vi "Untitled 1.vi"() -> ()   [LabVIEW 2013]
uses:
  <vilib>/MakerHub/LINX/Public/Peripherals/Digital/Digital Write 1 Chan.vi
  <vilib>/MakerHub/LINX/Public/Peripherals/Analog/Analog Read 1 Chan.vi
  <vilib>/MakerHub/LINX/Public/Peripherals/Digital/Digital Write N Chans.vi
  <vilib>/MakerHub/LINX/Public/Peripherals/Analog/Analog Read N Chans.vi
  <vilib>/MakerHub/LINX/Private/Local IO/LinxDigitalWrite.vi
  <vilib>/MakerHub/LINX/Public/Utilities/Check Channel.vi
  <vilib>/MakerHub/LINX/Private/Local IO/LinxAnalogRead.vi
  <vilib>/MakerHub/LINX/Public/Utilities/Open Serial.vi
  <vilib>/Utility/config.llb/Read Key (I32).vi
  <vilib>/Utility/config.llb/Read Key (Double).vi
  <vilib>/Utility/config.llb/Read Key (U32).vi
  <vilib>/Utility/config.llb/Write Key (U32).vi
  <vilib>/Utility/config.llb/Write Key (Double).vi
  <vilib>/MakerHub/LINX/Private/Utilties/Generate Error.vi
  <vilib>/express/express arith-compare/Formula/XNode/ExpressFormulaBlockNode.xnode
  <vilib>/MakerHub/LINX/LMH-LINX.lvlib
  <vilib>/Utility/config.llb/NI_LVConfig.lvlib
panel:
  out "Alarm":bool
  out "Relay":bool
  out "Moisture Value":dbl
  out "Alarm Pin":dbl
  out "Relay Pin":dbl
  out "Sensor Pin":dbl
  out "Critical Moisture Level":dbl
  out "Higher Moisture Level":dbl
  out "Lower Moisture Level":dbl
  in  "?":bool
  in  "Sensor":u8
  in  "higher moisture level":dbl
  in  "Relay":u8
  in  "critical moisture level":dbl
  in  "Alarm":u8
  in  "lower moisture level":dbl
  out "Moisture Level":dbl(slide) scale=0.0..100.0
  out "Waveform Chart":dbl(graph)
  in  "?":bool
  in  "Serial Port":refnum<visa-resource-name>="N/A"
  # "Automatic Plant Watering System"
  # "Pin Connections"
  # "Moisture Levels"
  # "Settings"
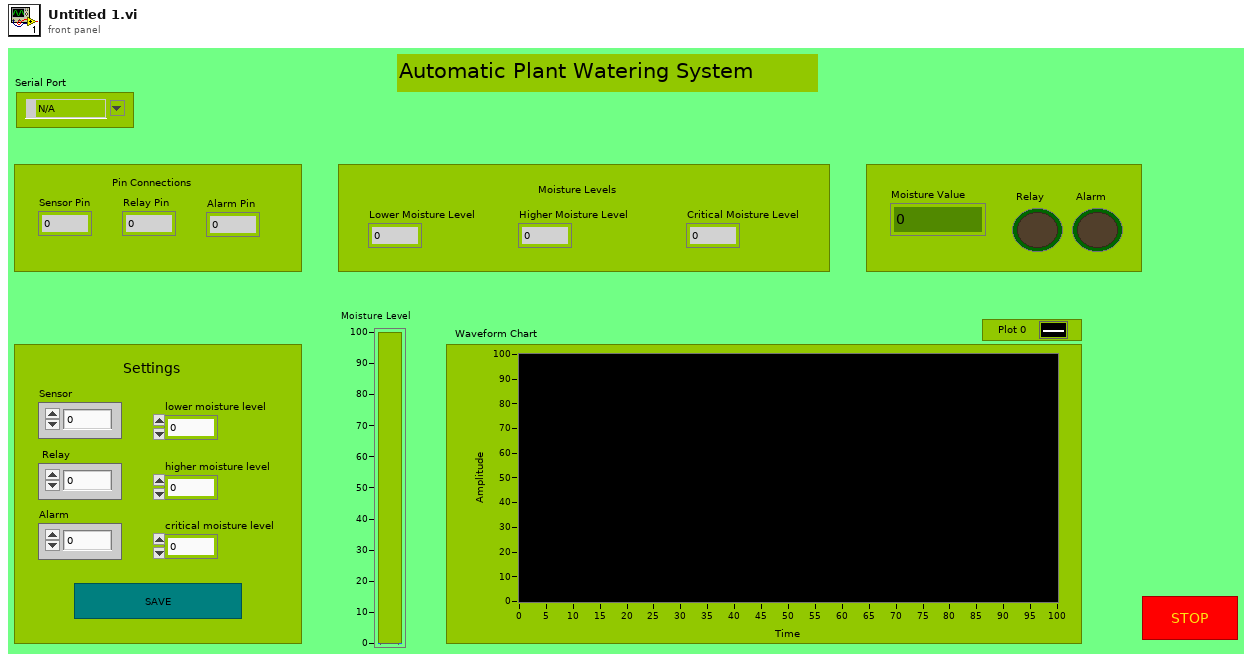
[diagram p1: front panel]
types:
  T1 = typedef "LMH-LINX.lvlib/LINX Ref.ctl" = cluster{"IO":T2, "Interface":T3, "LINX Device Config":T4}
  T2 = typedef "LMH-LINX.lvlib/Platform.ctl" = enum16{"Remote", "Local"}
  T3 = typedef "LMH-LINX.lvlib/Interface.ctl" = enum16{"Serial", "TCP"}
  T4 = typedef "LMH-LINX.lvlib/Device.lvlib/LINX Device Config.ctl" = cluster{"Interface":T3, "COM Port":refnum<visa-resource-name>, "TCP Configuration":T5, "Device Family":u8, "Device ID":u8, "Device Name":string, "TCP Ref":refnum<k5>, "Channels":T6}
  T5 = typedef "LMH-LINX.lvlib/Device.lvlib/TCP Config.ctl" = cluster{"IP Address":string, "Port":u16}
  T6 = typedef "LMH-LINX.lvlib/Channels.ctl" = cluster{"DI":u8[], "DO":u8[], "AI":u8[], "AO":u8[], "PWM":u8[], "QE":u8[], "UART":u8[], "I2C 2":u8[], "SPI":u8[], "CAN":u8[], "Servo":u8[], "AI Ref (V)":dbl, "AI Resolution (Bits)":u8, "AO Ref (V)":dbl, "AO Resolution (Bits)":u8}
  T7 = typedef "NI_LVConfig.lvlib/Config Data RefNum.ctl" = refnum<k1>
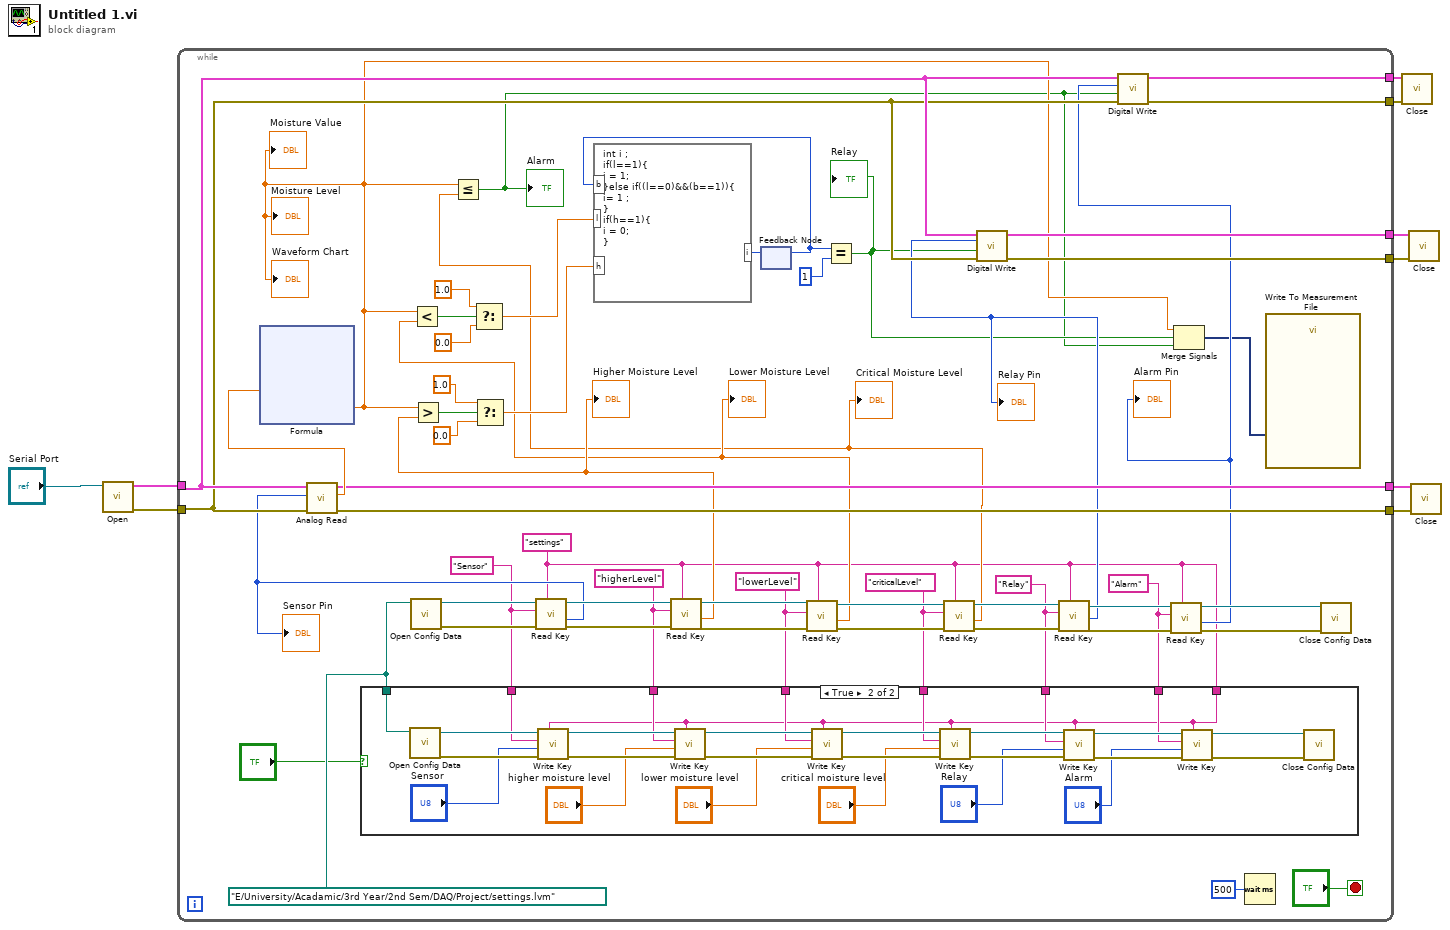
[diagram p0: block diagram]
diagram:
  n1 = call-poly <vilib>:"Open.vi"("Serial Port"="Serial Port") -> ("Error Out"=w6:errorcluster, "LINX Resource"=w7:T1)  [unwired: 8 in, 1 out]
  n2 = while {
    tunnel: [w62] -> w9
    tunnel: [w54] -> w8
    tunnel: w7 -> [w59]
    tunnel: w6 -> [w58]
    tunnel: [w61] -> w5
    tunnel: [w60] -> w4
    tunnel: [w57] -> w3
    tunnel: [w56] -> w2
    stop <- "?" stop-if-true
    w16 = "Alarm" ("key")
    w17 = "Relay" ("key")
    w18 = "criticalLevel" ("key")
    w19 = "lowerLevel" ("key")
    w20 = "higherLevel" ("key")
    w21 = "Sensor" ("key")
    w15 = "settings" ("section")
    w22 = path "E:/University/Acadamic/3rd Year/2nd Sem/DAQ/Project/settings.lvm" ("configuration file path")
    n3 = case shown="True" "?" {
      tunnel: w22 -> [_ w90]
      tunnel: w21 -> [_ w77]
      tunnel: w20 -> [_ w76]
      tunnel: w19 -> [_ w75]
      tunnel: w18 -> [_ w74]
      tunnel: w17 -> [_ w73]
      tunnel: w16 -> [_ w72]
      tunnel: w15 -> [_ w71]
      frame False {
      }
      frame True {
        n4 = call <vilib>:"Open Config Data.vi"("configuration file path"=w90) -> ("error out"=w91:errorcluster, "refnum"=w92:T7)  [unwired: 8 in, 1 out]
        n5 = call-poly <vilib>:"Write Key.vi"("section"=w71, "error in (no error)"=w91, "value"="Sensor", "key"=w77, "refnum"=w92) -> ("error out"=w88:errorcluster, "refnum out"=w89:T7)  [unwired: 4 in, 1 out]
        n6 = call-poly <vilib>:"Write Key.vi"("section"=w71, "error in (no error)"=w88, "value"="higher moisture level", "key"=w76, "refnum"=w89) -> ("error out"=w86:errorcluster, "refnum out"=w87:T7)  [unwired: 4 in, 1 out]
        n7 = call-poly <vilib>:"Write Key.vi"("section"=w71, "error in (no error)"=w86, "value"="lower moisture level", "key"=w75, "refnum"=w87) -> ("error out"=w84:errorcluster, "refnum out"=w85:T7)  [unwired: 4 in, 1 out]
        n8 = call-poly <vilib>:"Write Key.vi"("section"=w71, "error in (no error)"=w84, "value"="critical moisture level", "key"=w74, "refnum"=w85) -> ("error out"=w82:errorcluster, "refnum out"=w83:T7)  [unwired: 4 in, 1 out]
        n9 = call-poly <vilib>:"Write Key.vi"("section"=w71, "error in (no error)"=w82, "value"="Relay", "key"=w73, "refnum"=w83) -> ("error out"=w80:errorcluster, "refnum out"=w81:T7)  [unwired: 4 in, 1 out]
        n10 = call-poly <vilib>:"Write Key.vi"("section"=w71, "error in (no error)"=w80, "value"="Alarm", "key"=w72, "refnum"=w81) -> ("error out"=w78:errorcluster, "refnum out"=w79:T7)  [unwired: 4 in, 1 out]
        n11 = call <vilib>:"Close Config Data.vi"("error in (no error)"=w78, "refnum"=w79) -> ()  [unwired: 8 in, 2 out]
      }
    }
    n12 = call <vilib>:"Open Config Data.vi"("configuration file path"=w22) -> ("error out"=w43:errorcluster, "refnum"=w42:T7)  [unwired: 8 in, 1 out]
    n13 = call-poly <vilib>:"Read Key.vi"("section"=w15, "error in (no error)"=w43, "key"=w21, "refnum"=w42) -> ("error out"=w40:errorcluster, "value"=w28:i32, "refnum out"=w41:T7)  [unwired: 4 in, 1 out]
    "Sensor Pin" <- w28
    n14 = call-poly <vilib>:"Analog Read.vi"("Error In"=w58, "Analog Channel"=w28, "LINX Resource"=w59) -> ("Error Out"=w62:errorcluster, "Voltage"=w55:dbl, "LINX Resource"=w54:T1)  [unwired: 5 in, 1 out]
    n15 = xnode "Formula"("X1"=w55) -> ("Result"=w12:dbl)  [unwired: 1 in, 1 out]
    "Waveform Chart" <- w12
    "Moisture Value" <- w12
    "Moisture Level" <- w12
    n16 = call-poly <vilib>:"Read Key.vi"("section"=w15, "error in (no error)"=w40, "key"=w20, "refnum"=w41) -> ("error out"=w38:errorcluster, "value"=w27:dbl, "refnum out"=w39:T7)  [unwired: 4 in, 1 out]
    "Higher Moisture Level" <- w27
    n17 = Greater?(x=w12, y=w27) -> (0:w48:bool)
    n18 = Select(t=1.0, s=w48, f=0.0) -> (s? t:f=w47:dbl)
    n19 = feedback #1() -> (w45:i32)  [unwired: 1 in]
    n20 = call-poly <vilib>:"Read Key.vi"("section"=w15, "error in (no error)"=w38, "key"=w19, "refnum"=w39) -> ("error out"=w36:errorcluster, "value"=w26:dbl, "refnum out"=w37:T7)  [unwired: 4 in, 1 out]
    "Lower Moisture Level" <- w26
    n21 = Less?(x=w12, y=w26) -> (x < y?=w53:bool)
    n22 = Select(t=1.0, s=w53, f=0.0) -> (s? t:f=w33:dbl)
    n23 = formula code="int i ;\nif(l==1){\ni = 1;\n}else if((l==0)&&(b==1)){\ni= 1 ;\n}\nif(h==1){\ni = 0;\n}"("l"=w33, "h"=w47, "b"=w45) -> ("i"=w46:i32)
    n24 = feedback-in #1(w46) -> ()
    n25 = Equal?(x=w45, y=1) -> (x = y?=w11:bool)
    "Relay" <- w11
    n26 = call-poly <vilib>:"Read Key.vi"("section"=w15, "error in (no error)"=w36, "key"=w18, "refnum"=w37) -> ("error out"=w34:errorcluster, "value"=w25:dbl, "refnum out"=w35:T7)  [unwired: 4 in, 1 out]
    "Critical Moisture Level" <- w25
    n27 = Less Or Equal?(x=w12, y=w25) -> (x <= y?=w10:bool)
    "Alarm" <- w10
    n28 = call-poly <vilib>:"Read Key.vi"("section"=w15, "error in (no error)"=w34, "key"=w17, "refnum"=w35) -> ("error out"=w31:errorcluster, "value"=w24:u32, "refnum out"=w32:T7)  [unwired: 4 in, 1 out]
    "Relay Pin" <- w24
    n29 = call-poly <vilib>:"Digital Write.vi"("Error In"=w58, "Output Value"=w11, "DO Channel"=w24, "LINX Resource"=w59) -> ("Error Out"=w56:errorcluster, "LINX Resource"=w57:T1)  [unwired: 6 in]
    n30 = call-poly <vilib>:"Read Key.vi"("section"=w15, "error in (no error)"=w31, "key"=w16, "refnum"=w32) -> ("error out"=w30:errorcluster, "value"=w23:u32, "refnum out"=w29:T7)  [unwired: 4 in, 1 out]
    "Alarm Pin" <- w23
    n31 = call-poly <vilib>:"Digital Write.vi"("Error In"=w58, "Output Value"=w10, "DO Channel"=w23, "LINX Resource"=w59) -> ("Error Out"=w61:errorcluster, "LINX Resource"=w60:T1)  [unwired: 6 in]
    n32 = Merge Signals(w12, w11, w10) -> (w13:dynamicdata)
    n33 = Wait (ms)(milliseconds to wait=u32 500) -> ()  [unwired: 1 out]
    n34 = call "Write To Measurement File"("Signals"=w13) -> ()  [unwired: 16 in, 3 out]
    n35 = call <vilib>:"Close Config Data.vi"("error in (no error)"=w30, "refnum"=w29) -> ()  [unwired: 8 in, 2 out]
  }
  n36 = call <vilib>:"Close.vi"("Error In"=w5, "LINX Resource"=w4) -> ()  [unwired: 9 in, 1 out]
  n37 = call <vilib>:"Close.vi"("Error In"=w2, "LINX Resource"=w3) -> ()  [unwired: 9 in, 1 out]
  n38 = call <vilib>:"Close.vi"("Error In"=w9, "LINX Resource"=w8) -> ()  [unwired: 9 in, 1 out]
